vi "Template_Write Index Set.vi"(9 "Values":T1[](array[typedef]), 11 "Indices":i32[](array[numeric])) -> ()   [LabVIEW 2010, in "Current Value Table.lvlib"]
doc: "This VI writes a set of data as defined by the GetIndices function. This VI can provide an order of magnitude increase in performance over a normal index write for sufficiently large data sets."
uses:
  Template_Datatype.ctl
  Type Defs/Memory Commands.ctl
  I32_Memory Block.vi
  Current Value Table.lvlib
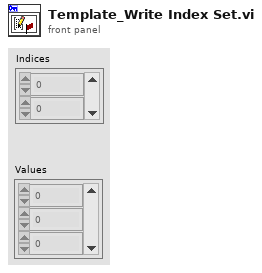
[diagram p1: front panel]
types:
  T1 = typedef "Template_Datatype.ctl" = i32
  T2 = typedef "Current Value Table.lvlib/Memory Commands.ctl" = enum16{"Init", "Add Data", "Read", "Read Group", "Read All", "Write", "Write Group", "Get Size"}
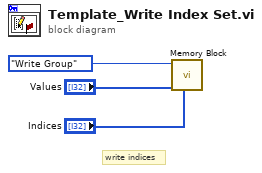
[diagram p0: block diagram]
diagram:
  # "write indices"
  n1 = call-poly "Memory Block.vi"("Group Indices"="Indices", "Data In"="Values", "Method"=Memory_Commands."Write Group") -> ()  [unwired: 6 in, 3 out]
